vi "Execute.vi"(8 "error in (no error)":errorcluster, 10 "Motor in":refnum<class "Motor.lvclass">, 11 "Wait in":refnum<class "Wait.lvclass">) -> (0 "error out":errorcluster, 1 "Status message":string, 2 "Motor out":refnum<class "Motor.lvclass">, 3 "Wait out":refnum<class "Wait.lvclass">)   [LabVIEW 2013, in "PowderDeposition.lvlib" / "Wait.lvclass"]
uses:
  Wait.lvclass
  Motor/Motor.lvclass
  Wait.lvclass/Wait.ctl
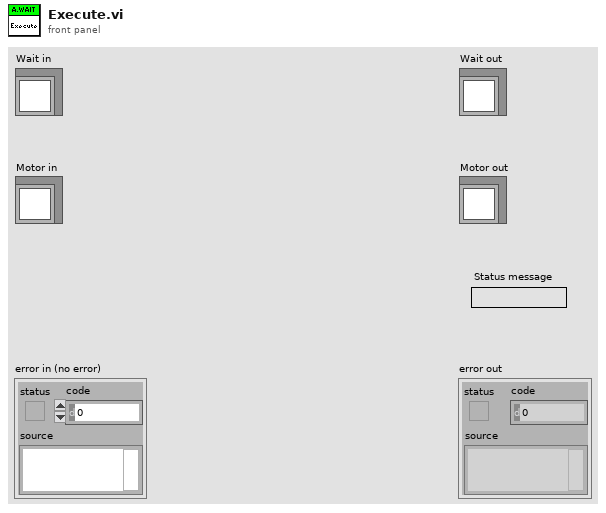
[diagram p1: front panel]
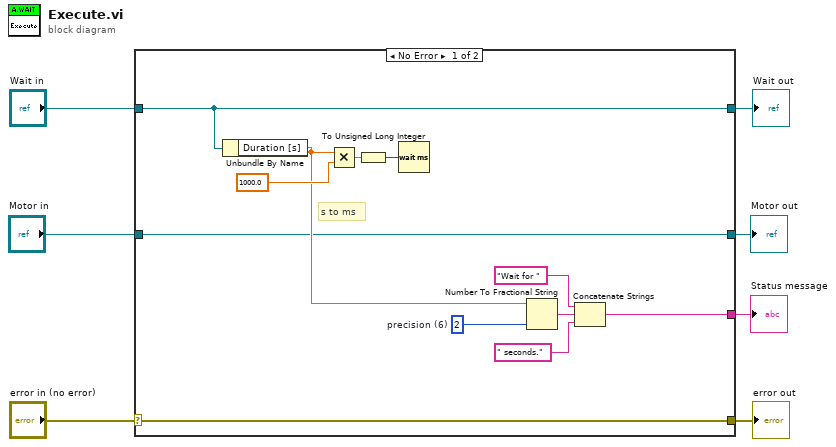
[diagram p0: block diagram]
diagram:
  n1 = case shown="No Error" "error in (no error)" {
    selector: "error in (no error)" -> [w19 w22]
    tunnel: [w19 w22] -> w6
    tunnel: [w8 w21] -> w4
    tunnel: "Wait in" -> [w8 w21]
    tunnel: [w9 _] -> w3
    tunnel: "Motor in" -> [w10 w20]
    tunnel: [w10 w20] -> w1
    frame No Error {
      w11 = i16 2  # precision (6)
      # "s to ms"
      n2 = Unbundle By Name(w8) -> ("Duration [s]"=w14:dbl)
      n3 = Multiply(x=w14, y=1000.0) -> (x*y=w18:dbl)
      n4 = To Unsigned Long Integer(number=w18) -> (unsigned 32bit integer=w16:u32)
      n5 = Wait (ms)(milliseconds to wait=w16) -> ()  [unwired: 1 out]
      n6 = Number To Fractional String(number=w14, precision (6)=w11) -> (F-format string=w15:string)  [unwired: 2 in]
      n7 = Concatenate Strings("Wait for ", w15, " seconds.") -> (w9:string)
    }
    frame Error {
    }
  }
  "error out" <- w6
  "Wait out" <- w4
  "Status message" <- w3
  "Motor out" <- w1
